vi "Global Strings.vi"() -> ()   [LabVIEW 2017, in "NI_Robotics_Configure Steering Frame.lvlib"]
uses:
  <vilib>/robotics/Dialog/Configure Steering Frame/NI_Robotics_Configure Steering Frame.lvlib
panel:
  in  "change steer type_F":string="Cancel"
  in  "change steer type_T":string="Change"
  in  "change steer type_msg":string="Changing the steering type will erase the current configuration."
  in  "picture tip strip":string
  in  "picture description":string
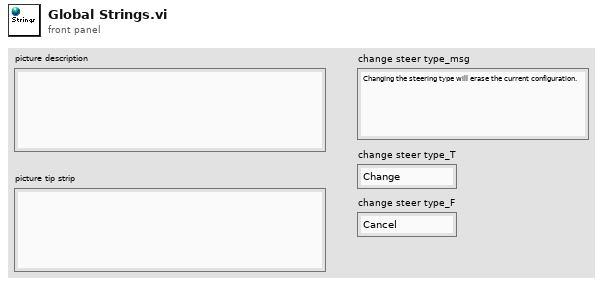
[diagram p1: front panel]
diagram:
